vi "Drive Motor Request Values.vi"(10 "Drive Motor Handle In":T1, 11 "Error In":errorcluster) -> (2 "Drive Motor Handle Out":T1, 3 "Error Out":errorcluster)   [LabVIEW 2021]
uses:
  Drive Motor Handle.ctl
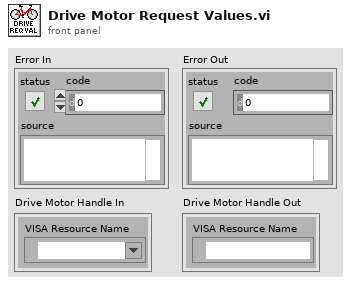
[diagram p1: front panel]
types:
  T1 = typedef "Drive Motor Handle.ctl" = cluster{"VISA Resource Name":refnum<visa-resource-name>}
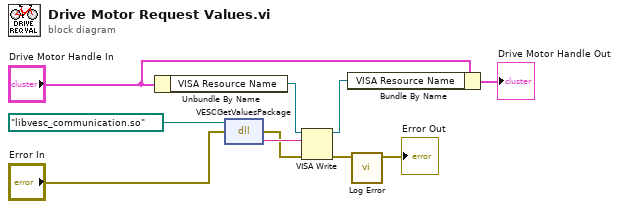
[diagram p0: block diagram]
diagram:
  n1 = Unbundle By Name("Drive Motor Handle In") -> ("VISA Resource Name"=w5:refnum<visa-resource-name>)
  n2 = dll-call lib="?" fn="VESCGetValuesPackage"(path in=path "libvesc_communication.so", error in="Error In") -> (error out=w1:errorcluster, "Package"=w7:string)  [unwired: 1 in, 1 out]
  n3 = VISA Write(VISA resource name=w5, write buffer=w7, error in (no error)=w1) -> (VISA resource name out=w4:refnum<visa-resource-name>, error out=w6:errorcluster)  [unwired: 1 out]
  n4 = Bundle By Name(cluster="Drive Motor Handle In", "VISA Resource Name"=w4) -> (→"Drive Motor Handle Out":T1)
  n5 = call "Log Error.vi"("Error In"=w6) -> ("Error Out"=→"Error Out":errorcluster)  [unwired: 10 in]
